vi "ClassAppData.Util_Load INI File.vi"(8 "error in":errorcluster, 9 "RmtFileSect":string[](array[string]), 10 "Input INI":path, 11 "Data In":variant) -> (0 "error out":errorcluster, 2 "Additional Cfg Files":path[](array[path]), 3 "Data Out":variant)   [LabVIEW 2024, in "EQMF.lvlib" / "Config Utils.lvlib" / "Class.AppData.lvclass"]
doc: "<B>AppData Class:</B>\nThe AppData class keeps track of a library of data items that are used by an application. These data items have a name (text string) and value that can be any data type. \n\nThis VI is an internal utility that loads data for INI files and outputs a list of additional config files that were referenced by the INI file.\n\nINPUTS:\n<B>Input INI </B> - This contains the path to the INI file to read data items from.\n<B>Data In</B> - The is a variant contain attributes that make up a data library.\n<B>RmtFileSect</B> - The is a list of names of sections that contain paths to additional configuration files.\n\nOUTPUTS:\n<B>Data In</B> - The is a variant contain attributes that make up a data library. It contains the Data In items merged with any new items read from the Input INI file.\n<B>RmtFileSect</B> - The is a list of names of sections that contain paths to additional configuration files."
uses:
  Class.AppData.lvclass
  <vilib>/Utility/config.llb/Read Key (String).vi
  <vilib>/Utility/config.llb/NI_LVConfig.lvlib
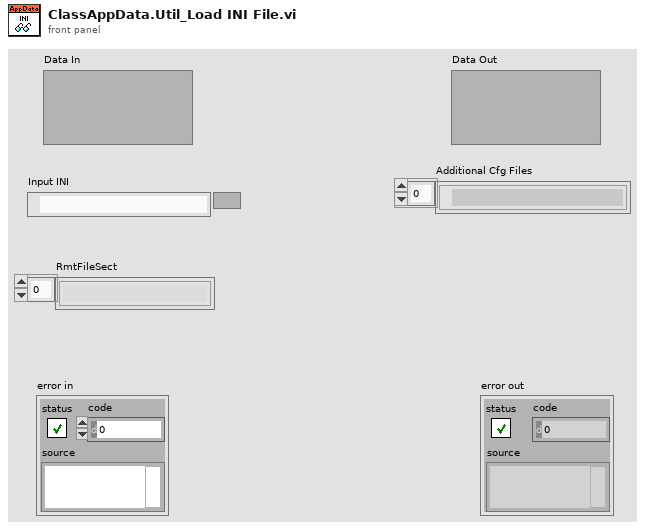
[diagram p1: front panel]
types:
  T1 = cluster{"CurrentFile":path, "Files":path[], "RmtFileSect":string[], "Error":errorcluster, "AddedFiles":path[], "FileCnt":i32}
  T2 = typedef "NI_LVConfig.lvlib/Config Data RefNum.ctl" = refnum<k1>
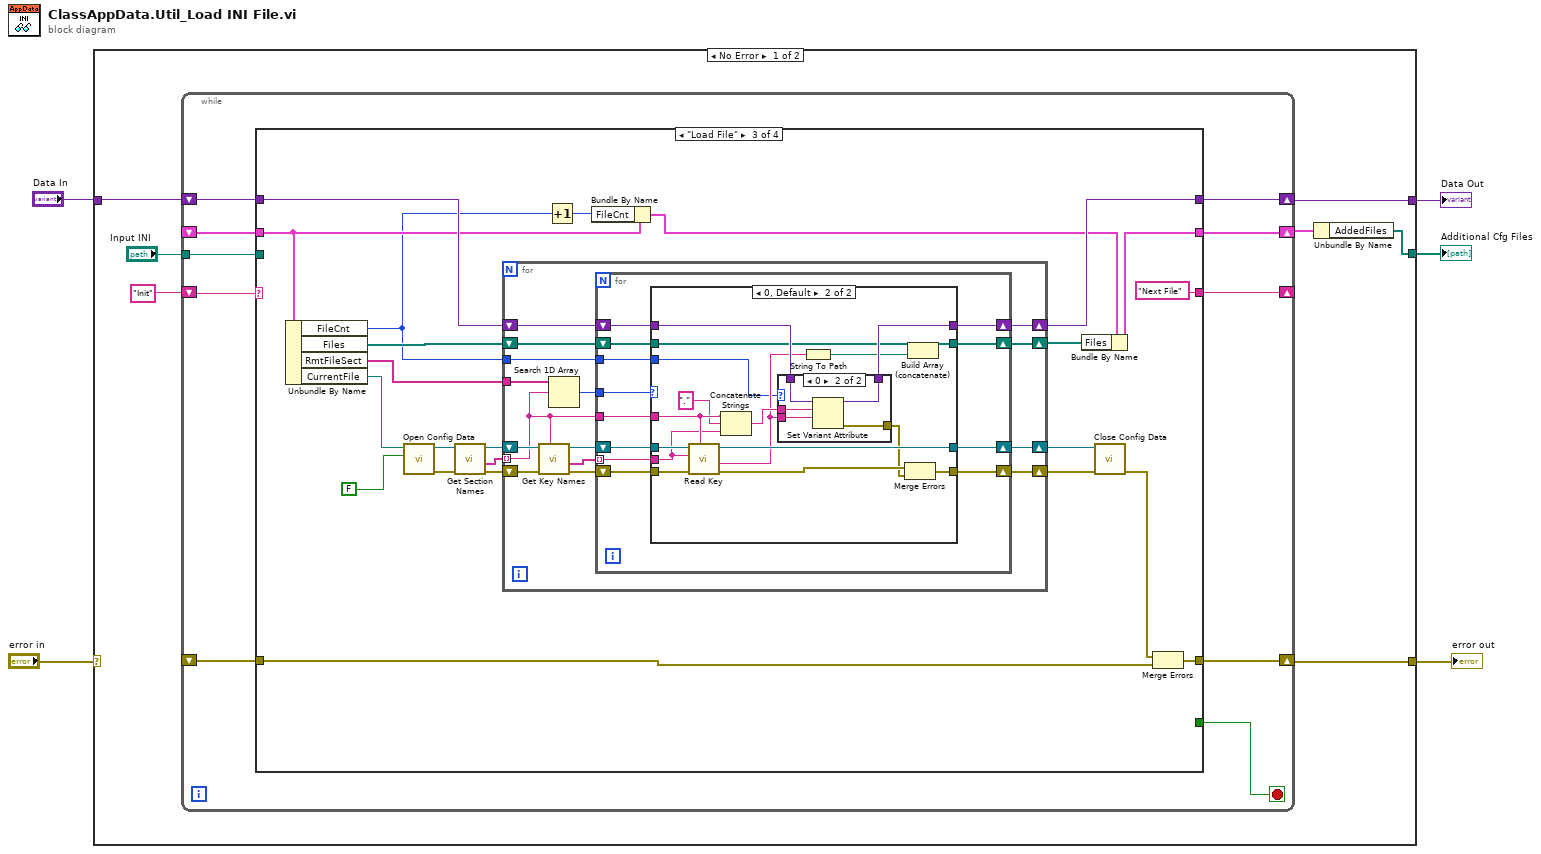
[diagram p0: block diagram]
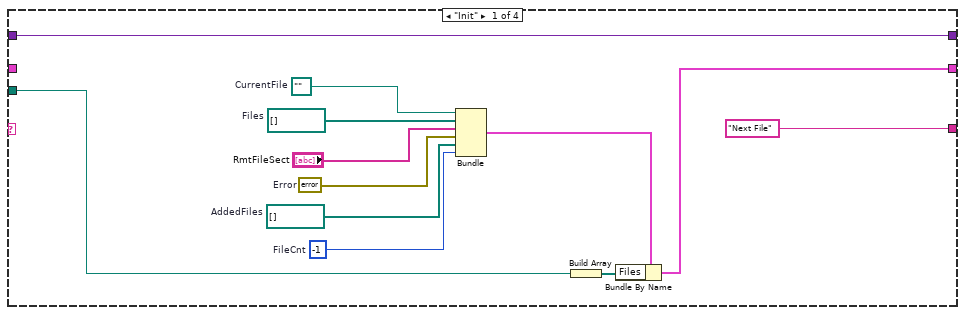
[diagram p2: hidden frame]
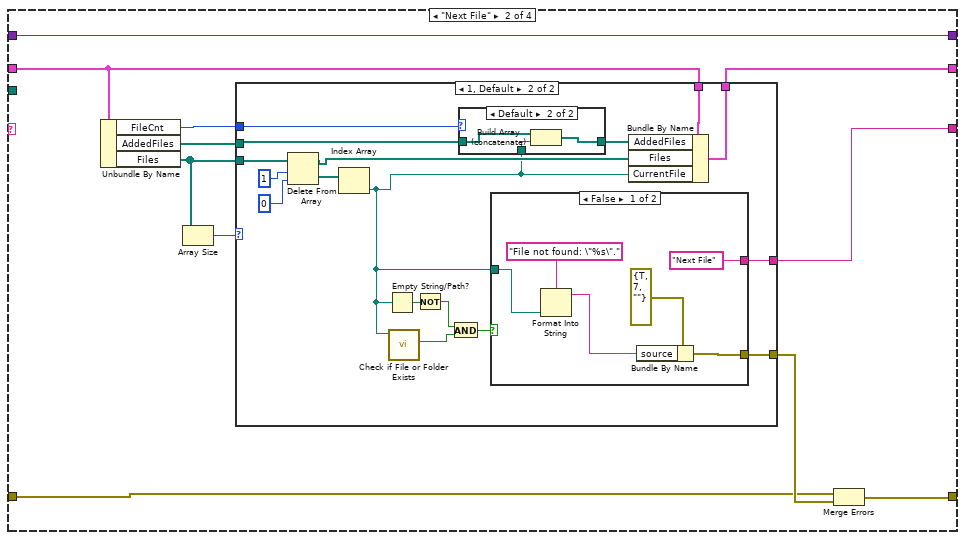
[diagram p3: hidden frame]
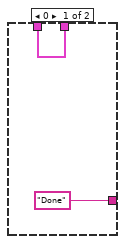
[diagram p4: hidden frame]
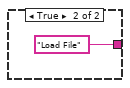
[diagram p6: hidden frame]
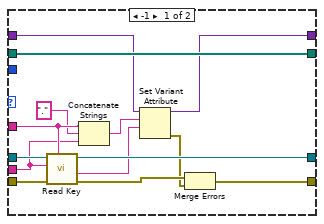
[diagram p7: hidden frame]
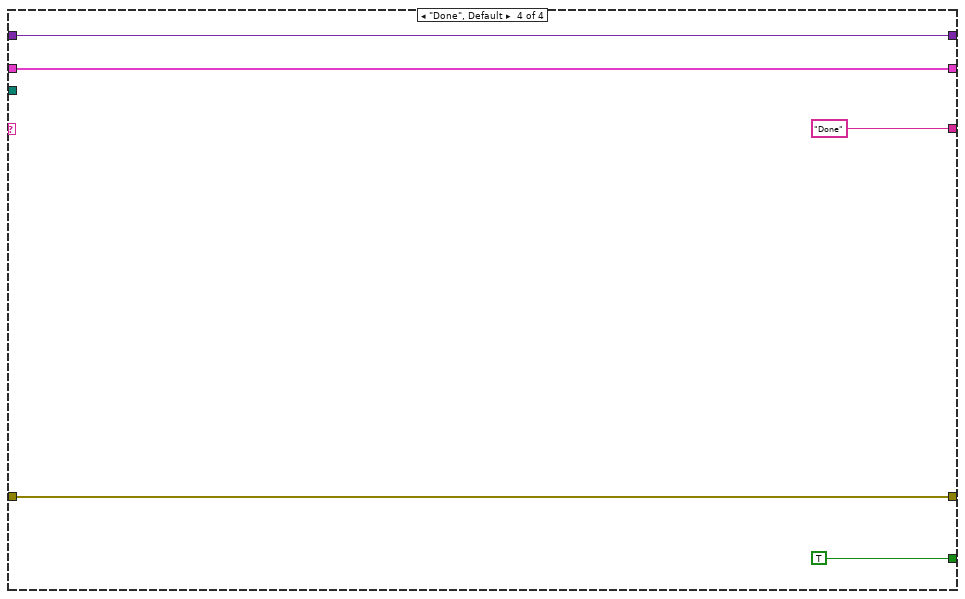
[diagram p9: hidden frame]
diagram:
  n1 = case shown="No Error" "error in" {
    selector: "error in" -> [_ w169]
    tunnel: [w9 w169] -> w4
    tunnel: [w8 w168] -> w2
    tunnel: "Data In" -> [w11 w168]
    tunnel: [w6 _] -> w1
    frame No Error {
      n2 = while {
        shift-right: [w21] -> _
        shift-left: "Init" -> [w18]
        shift-right: [w22] -> w7
        shift-left: _ -> [w17]
        shift-right: [w19] -> w8
        shift-left: w11 -> [w20]
        shift-right: [w15] -> w9
        shift-left: _ -> [w14]
        tunnel: "Input INI" -> [w13]
        stop <- w16 stop-if-true
        n3 = case shown="\"Load File\"" w18 {
          tunnel: [w30 w41 w85 w165] -> w22
          tunnel: ["Next File" w40 "Next File" "Done"] -> w21
          tunnel: w20 -> [w28 w45 w81 w163]
          tunnel: [w28 w45 w80 w163] -> w19
          tunnel: w17 -> [_ w42 w79 w165]
          tunnel: [_ _ _ TRUE] -> w16
          tunnel: [_ w39 w84 w164] -> w15
          tunnel: w14 -> [_ w37 w82 w164]
          tunnel: w13 -> [w24 _ _ _]
          frame "Init" {
            w23 = -1  # FileCnt
            w25 = path[] []  # AddedFiles
            w26 = path ""  # CurrentFile
            w27 = errorcluster {"status"=FALSE, "code"=0, "source"=""}  # Error
            w34 = path[] []  # Files
            n4 = Bundle("CurrentFile"=w26, "Files"=w34, "RmtFileSect"="RmtFileSect", "Error"=w27, "AddedFiles"=w25, "FileCnt"=w23) -> (w32:T1)  [unwired: 1 in]
            n5 = Build Array(w24) -> (w31:path[])
            n6 = Bundle By Name(cluster=w32, "Files"=w31) -> (w30:T1)
          }
          frame "Next File" {
            n7 = Unbundle By Name(w42) -> ("FileCnt"=w35:i32, "AddedFiles"=w36:path[], "Files"=w44:path[])
            n8 = Array Size(array=w44) -> (size(s)=w43:i32)
            n9 = case shown="1, Default" w43 {
              tunnel: w44 -> [_ w61]
              tunnel: w42 -> [w47 w60]
              tunnel: [w47 w58] -> w41
              tunnel: ["Done" w53] -> w40
              tunnel: [_ w52] -> w38
              tunnel: w36 -> [_ w51]
              tunnel: w35 -> [_ w48]
              frame 0 {
              }
              frame 1, Default {
                n10 = Delete From Array(array=w61, length=1, index=0 ("length")) -> (deleted portion=w62:path[], array with subset deleted=w59:path[])
                n11 = Index Array(array=w62) -> (element=w49:path)  [unwired: 1 in]
                n12 = Empty String/Path?(string/path=w49) -> (empty?=w57:bool)
                n13 = call <vilib>:"Check if File or Folder Exists.vi"("path"=w49) -> ("file or folder exists?"=w55:bool)  [unwired: 8 in, 2 out]
                n14 = Not(x=w57) -> (.not. x?=w56:bool)
                n15 = And(x=w56, y=w55) -> (x .and. y?=w54:bool)
                n16 = case shown="Default" w48 {
                  tunnel: w51 -> [w65 w68]
                  tunnel: [w65 w67] -> w50
                  tunnel: w49 -> [_ w66]
                  frame 0 {
                  }
                  frame Default {
                    n17 = Build Array (concatenate)(w68, w66) -> (w67:path[])
                  }
                }
                n18 = case shown="False" w54 {
                  tunnel: w49 -> [w73 _]
                  tunnel: ["Next File" "Load File"] -> w53
                  tunnel: [w69 _] -> w52
                  frame False {
                    n19 = Format Into String(format string="File not found: \"%s\".", w73) -> (resulting string=w70:string)  [unwired: 2 in, 1 out]
                    n20 = Bundle By Name(cluster=errorcluster {"status"=TRUE, "code"=7, "source"=""} ("error constant"), "source"=w70) -> (w69:errorcluster)
                  }
                  frame True {
                  }
                }
                n21 = Bundle By Name(cluster=w60, "AddedFiles"=w50, "Files"=w59, "CurrentFile"=w49) -> (w58:T1)
              }
            }
            n22 = Merge Errors(w37, w38) -> (w39:errorcluster)
          }
          frame "Load File" {
            n23 = Unbundle By Name(w79) -> ("FileCnt"=w76:i32, "Files"=w88:path[], "RmtFileSect"=w87:string[], "CurrentFile"=w96:path)
            n24 = call <vilib>:"Open Config Data.vi"("create file if necessary (T)"=FALSE, "configuration file path"=w96) -> ("error out"=w91:errorcluster, "refnum"=w92:T2)  [unwired: 7 in, 1 out]
            n25 = call <vilib>:"Get Section Names.vi"("error in (no error)"=w91, "refnum"=w92) -> ("error out"=w93:errorcluster, "section names"=w95:string[], "refnum out"=w94:T2)  [unwired: 7 in]
            n26 = for {
              tunnel: w95 -> [w102] mode=indexing
              shift-right: [w108] -> w89
              shift-left: w93 -> [w113]
              shift-right: [w107] -> w90
              shift-left: w94 -> [w112]
              shift-right: [w104] -> w86
              shift-left: w88 -> [w106]
              tunnel: w87 -> [w105]
              shift-right: [w101] -> w80
              shift-left: w81 -> [w100]
              tunnel: w76 -> [w99]
              n27 = call <vilib>:"Get Key Names.vi"("section"=w102, "error in (no error)"=w113, "refnum"=w112) -> ("error out"=w110:errorcluster, "key names"=w109:string[], "refnum out"=w111:T2)  [unwired: 5 in, 1 out]
              n28 = Search 1D Array(1D array=w105, element=w102) -> (index of element=w103:i32)  [unwired: 1 in]
              n29 = for {
                tunnel: w109 -> [w119] mode=indexing
                tunnel: w102 -> [w123]
                shift-right: [w122] -> w108
                shift-left: w110 -> [w124]
                shift-right: [w121] -> w107
                shift-left: w111 -> [w125]
                shift-right: [w118] -> w104
                shift-left: w106 -> [w120]
                tunnel: w103 -> [w117]
                shift-right: [w116] -> w101
                shift-left: w100 -> [w115]
                tunnel: w99 -> [w114]
                n30 = case shown="0, Default" w117 {
                  tunnel: w125 -> [w139 w156]
                  tunnel: w124 -> [w138 w155]
                  tunnel: w123 -> [w135 w153]
                  tunnel: w119 -> [w134 w152]
                  tunnel: [w128 w147] -> w122
                  tunnel: [w137 w154] -> w121
                  tunnel: w120 -> [w136 w144]
                  tunnel: [w136 w142] -> w118
                  tunnel: w115 -> [w130 w149]
                  tunnel: [w129 w148] -> w116
                  tunnel: w114 -> [_ w140]
                  frame -1 {
                    n31 = call-poly <vilib>:"Read Key.vi"("section"=w135, "error in (no error)"=w138, "key"=w134, "refnum"=w139) -> ("error out"=w127:errorcluster, "value"=w131:string, "refnum out"=w137:T2)  [unwired: 4 in, 1 out]
                    n32 = Concatenate Strings(w135, ".", w134) -> (w132:string)
                    n33 = Set Variant Attribute(Variant=w130, name=w132, value=w131) -> (Variant out=w129:variant, error out=w126:errorcluster)  [unwired: 1 in, 1 out]
                    n34 = Merge Errors(w127, w126) -> (w128:errorcluster)
                  }
                  frame 0, Default {
                    n35 = call-poly <vilib>:"Read Key.vi"("section"=w153, "error in (no error)"=w155, "key"=w152, "refnum"=w156) -> ("error out"=w146:errorcluster, "value"=w141:string, "refnum out"=w154:T2)  [unwired: 4 in, 1 out]
                    n36 = Concatenate Strings(w153, ".", w152) -> (w150:string)
                    n37 = case shown="0" w140 {
                      tunnel: w150 -> [_ w162]
                      tunnel: w149 -> [w157 w161]
                      tunnel: [w157 w160] -> w148
                      tunnel: [_ w159] -> w145
                      tunnel: w141 -> [_ w158]
                      frame Default {
                      }
                      frame 0 {
                        n38 = Set Variant Attribute(Variant=w161, name=w162, value=w158) -> (Variant out=w160:variant, error out=w159:errorcluster)  [unwired: 1 in, 1 out]
                      }
                    }
                    n39 = String To Path(string=w141) -> (path=w143:path)
                    n40 = Merge Errors(w146, w145) -> (w147:errorcluster)
                    n41 = Build Array (concatenate)(w144, w143) -> (w142:path[])
                  }
                }
              }
            }
            n42 = Increment(x=w76) -> (x+1=w77:i32)
            n43 = Bundle By Name(cluster=w79, "FileCnt"=w77) -> (w78:T1)
            n44 = Bundle By Name(cluster=w78, "Files"=w86) -> (w85:T1)
            n45 = call <vilib>:"Close Config Data.vi"("error in (no error)"=w89, "refnum"=w90) -> ("error out"=w83:errorcluster)  [unwired: 8 in, 1 out]
            n46 = Merge Errors(w83, w82) -> (w84:errorcluster)
          }
          frame "Done", Default {
          }
        }
      }
      n47 = Unbundle By Name(w7) -> ("AddedFiles"=w6:path[])
    }
    frame Error {
    }
  }
  "error out" <- w4
  "Data Out" <- w2
  "Additional Cfg Files" <- w1
